vi "InitScan.vi"(9 "Spectral Channels Bool":bool[](array[boolean]), 10 "Spectrometer wavelengths (All)":sgl[][](array[numeric]), 11 "Spectral Channels (All)":i32[](array[numeric])) -> (2 "Spectrometer wavelengths (filtered)":sgl[][](array[numeric]), 3 "Spectral Channels (filtered)":i32[](array[numeric]))   [LabVIEW 2012]
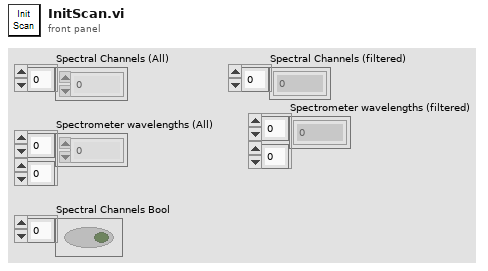
[diagram p1: front panel]
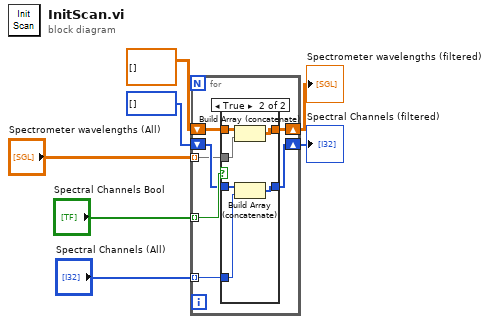
[diagram p0: block diagram]
diagram:
  n1 = for {
    tunnel: "Spectral Channels Bool" -> [w14] mode=indexing
    tunnel: "Spectral Channels (All)" -> [w13] mode=indexing
    shift-right: [w12] -> w5
    shift-left: i32[] [] -> [w11]
    tunnel: "Spectrometer wavelengths (All)" -> [w10] mode=indexing
    shift-right: [w8] -> w1
    shift-left: sgl[][] [] -> [w9]
    n2 = case shown="True" w14 {
      tunnel: w13 -> [_ w22]
      tunnel: [w16 w21] -> w12
      tunnel: w11 -> [w16 w20]
      tunnel: w10 -> [_ w19]
      tunnel: [w15 w18] -> w8
      tunnel: w9 -> [w15 w17]
      frame False {
      }
      frame True {
        n3 = Build Array (concatenate)(w17, w19) -> (w18:sgl[][])
        n4 = Build Array (concatenate)(w20, w22) -> (w21:i32[])
      }
    }
  }
  "Spectral Channels (filtered)" <- w5
  "Spectrometer wavelengths (filtered)" <- w1
